vi "Time domain Tx-TF Correction.vi"(7 "Normalize to TF":bool=TRUE, 10 "window":T1=1 items=["Rectangle"=0, "Hanning"=1, "Hamming"=2, "Blackman-Harris"=3, "Exact Blackman"=4, "Blackman"=5, "Flat Top"=6, "4 Term B-Harris "=7, "7 Term B-Harris"=8, "Low Sidelobe"=9, "Blackman Nuttall"=11, "Triangle"=30, "Bartlett-Hanning"=31, "Bohman"=32, "Parzen"=33, "Welch"=34, "Kaiser"=60, "Dolph-Chebyshev"=61, "Gaussian"=62], 11 "Tx Waveform":waveform(dbl)={"t0"=timestamp(3728232981.5205336 s since 1904-01-01), "dt"=9.9999999999997e-07, "Y"=array[20000 elements], "attributes"=variant("NI_ChannelName"=variant(string "H1/ai7"), "NI_UnitDescription"=variant(string "Volts"))}) -> (0 "Rx FFT _NoCorrect":cluster{"f0":dbl, "df":dbl, "magnitude":dbl[]}(graph), 1 "Waveform Graph":cluster{"f0":dbl, "df":dbl, "magnitude":dbl[]}(graph), 2 "TF units from loaded file":string, 3 "TF Corr Rx FFT complex":T2, 4 "IMon magnitude":dbl, 6 "THD":dbl)   [LabVIEW 2021]
uses:
  <vilib>/Analysis/4window.llb/windowTd.ctl
  <vilib>/measure/maspectr.llb/Power Spectrum and PSD Export Mode.ctl
  <vilib>/Analysis/2dsp.llb/Inverse Real FFT.vi
  <vilib>/measure/maspectr.llb/FFT Spectrum (Mag-Phase) for 1 Chan.vi
  <vilib>/measure/maspectr.llb/FFT Power Spectrum and PSD for 1 Chan.vi
  MPS_Labview/MPS_global_variables.vi
  <vilib>/measure/NI_MAPro.lvlib
  <vilib>/Analysis/NI_AALPro.lvlib
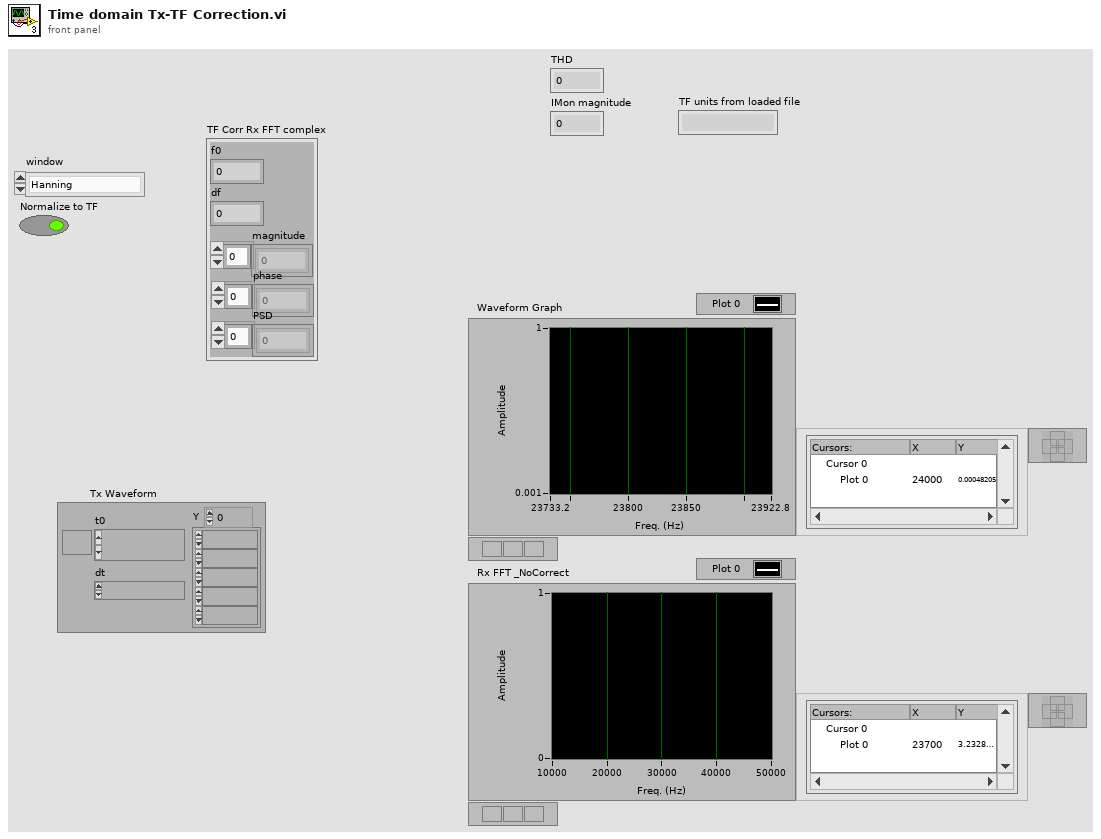
[diagram p1: front panel]
types:
  T1 = typedef "NI_AALPro.lvlib/windowTd.ctl" = u32
  T2 = cluster{"f0":dbl, "df":dbl, "magnitude":dbl[], "phase":dbl[], "PSD":dbl[]}
  T3 = cluster{"sample rate":dbl, "Transmit frequency":dbl, "Transmit amplitude":dbl, "sample rate digital out":dbl, "TX cycles":i32, "sample rate DAQ1":dbl, "Receive frequency":dbl, "Receive range":dbl, "TX harmonics":dbl[]}
  T4 = typedef "NI_MAPro.lvlib/Power Spectrum and PSD Export Mode.ctl" = u16
  T5 = cluster{"sample rate":dbl, "Tx freq":dbl, "Tx amp":dbl, "Tx cycles\nSpectroscopy":dbl, "Bias amp":dbl, "Bias freq":dbl, "Receive range":dbl, "Bias Periods\nMagnetometry":dbl, "Tx Freq Division Factor":dbl, "Drive Periods per Bias":dbl, "TX harmonics":dbl[]}
  T6 = cluster{"f0":dbl, "df":dbl, "magnitude":dbl[], "phase":dbl[], dbl[]}
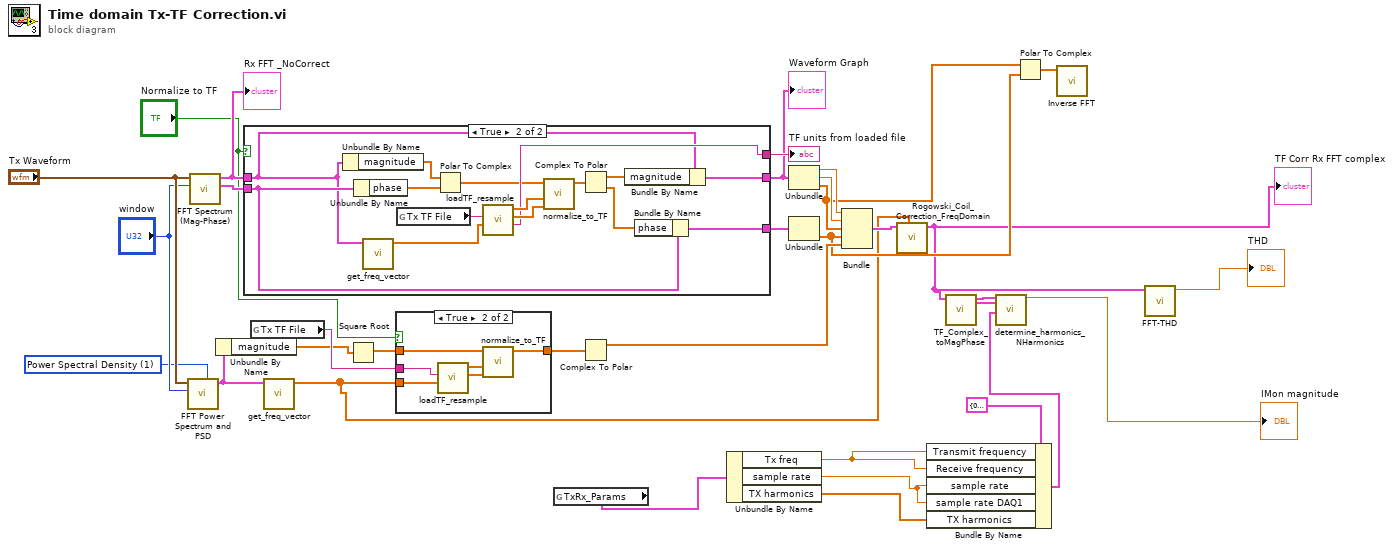
[diagram p0: block diagram]
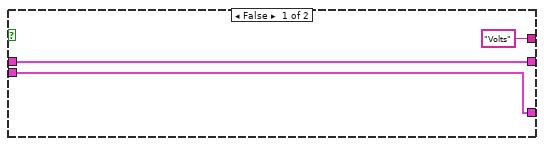
[diagram p3: hidden frame]
diagram:
  w23 = T4 1 items=["Power Spectrum", "Power Spectral Density"] ("export mode")
  n1 = call-poly <vilib>:"FFT Power Spectrum and PSD.vi"("export mode"=w23, "window"="window", "time signal"="Tx Waveform") -> ("Power Spectrum / PSD"=w26:cluster{"f0":dbl, "df":dbl, "magnitude":dbl[]})  [unwired: 5 in, 3 out]
  n2 = call-poly <vilib>:"FFT Spectrum (Mag-Phase).vi"("window"="window", "time signal"="Tx Waveform") -> ("phase"=w33:cluster{"f0":dbl, "df":dbl, "phase":dbl[]}, "magnitude"=w31:cluster{"f0":dbl, "df":dbl, "magnitude":dbl[]})  [unwired: 5 in, 3 out]
  "Rx FFT _NoCorrect" <- w31
  n3 = Unbundle By Name(w26) -> ("magnitude"=w20:dbl[])
  n4 = case shown="True" "Normalize to TF" {
    tunnel: w33 -> [w35 w46]
    tunnel: ["Volts" ("TF units from loaded file") w43] -> w32
    tunnel: w31 -> [w36 w37]
    tunnel: [w36 w39] -> w15
    tunnel: [w35 w38] -> w14
    frame False {
    }
    frame True {
      n5 = Unbundle By Name(w37) -> ("magnitude"=w48:dbl[])
      n6 = Unbundle By Name(w46) -> ("phase"=w47:dbl[])
      n7 = call "get_freq_vector.vi"("FFT magnitude"=w37) -> ("Freq array"=w49:dbl[])  [unwired: 10 in]
      n8 = global read "MPS_global_variables.vi" "Tx TF File"() -> (w44:string)
      n9 = Polar To Complex(1:w47, 2:w48) -> (0:w41:cdb[])
      n10 = call "loadTF_resample.vi"("desired freqs"=w49, "mat file name"=w44) -> ("TF units from loaded file"=w43:string, "output TF phase"=w51:dbl[], "output TF mag"=w50:dbl[])  [unwired: 7 in]
      n11 = call "normalize_to_TF.vi"("TF phase"=w51, "TF mag"=w50, "signal (can be complex)"=w41) -> ("signal normalized to TF (can be complex)"=w40:cdb[])  [unwired: 8 in]
      n12 = Complex To Polar(r * e^(i*theta)=w40) -> (r=w42:dbl[], theta=w45:dbl[])
      n13 = Bundle By Name(cluster=w37, "magnitude"=w42) -> (w39:cluster{"f0":dbl, "df":dbl, "magnitude":dbl[]})
      n14 = Bundle By Name(cluster=w46, "phase"=w45) -> (w38:cluster{"f0":dbl, "df":dbl, "phase":dbl[]})
    }
  }
  "TF units from loaded file" <- w32
  "Waveform Graph" <- w15
  n15 = global read "MPS_global_variables.vi" "Tx TF File"() -> (w27:string)
  n16 = call "get_freq_vector.vi"("FFT magnitude"=w26) -> ("Freq array"=w1:dbl[])  [unwired: 10 in]
  n17 = Square Root(x=w20) -> (sqrt(x)=w21:dbl[])
  n18 = case shown="True" "Normalize to TF" {
    tunnel: [w52 w58] -> w28
    tunnel: w27 -> [_ w57]
    tunnel: w1 -> [_ w56]
    tunnel: w21 -> [w52 w53]
    frame False {
    }
    frame True {
      n19 = call "loadTF_resample.vi"("desired freqs"=w56, "mat file name"=w57) -> ("output TF phase"=w54:dbl[], "output TF mag"=w55:dbl[])  [unwired: 7 in, 1 out]
      n20 = call "normalize_to_TF.vi"("TF phase"=w54, "TF mag"=w55, "signal (can be complex)"=w53) -> ("signal normalized to TF (can be complex)"=w58:cdb[])  [unwired: 8 in]
    }
  }
  n21 = global read "MPS_global_variables.vi" "TxRx_Params"() -> (w13:T5)
  n22 = Complex To Polar(r * e^(i*theta)=w28) -> (r=w25:dbl[])  [unwired: 1 out]
  n23 = Unbundle By Name(w13) -> ("Tx freq"=w11:dbl, "sample rate"=w10:dbl, "TX harmonics"=w9:dbl[])
  n24 = Unbundle(w15) -> ("f0"=w19:dbl, "df"=w30:dbl, "magnitude"=w18:dbl[])
  n25 = Unbundle(w14) -> ("phase"=w17:dbl[])  [unwired: 2 out]
  n26 = Bundle("f0"=w19, "df"=w30, "magnitude"=w18, "phase"=w17, w25) -> (w5:T6)  [unwired: 1 in]
  n27 = call "Rogowski_Coil_Correction_FreqDomain.vi"("Freq array"=w1, "Raw IMon FFT"=w5) -> ("TF Corr IMon FFT"=w4:T2)  [unwired: 8 in, 1 out]
  "TF Corr Rx FFT complex" <- w4
  n28 = Bundle By Name(cluster=T3 {"sample rate"=0.0, "Transmit frequency"=0.0, "Transmit amplitude"=0.0, "sample rate digital out"=0.0, "TX cycles"=0, "sample rate DAQ1"=0.0, "Receive frequency"=0.0, "Receive range"=0.0, "TX harmonics"=[]} ("TxRxParams"), "Transmit frequency"=w11, "Receive frequency"=w11, "sample rate"=w10, "sample rate DAQ1"=w10, "TX harmonics"=w9) -> (w8:T3)
  n29 = call "TF_Complex_toMagPhase.vi"("TF Corr Rx FFT Mag"=w4) -> ("TF Phase"=w2:cluster{"f0":dbl, "df":dbl, "magnitude":dbl[]}, "TF Mag"=w3:cluster{"f0":dbl, "df":dbl, "magnitude":dbl[]})  [unwired: 4 in, 5 out]
  n30 = call "determine_harmonics_NHarmonics.vi"("FFT magnitude"=w3, "FFT phase"=w2, "TxRxParams"=w8) -> ("RX magnitude"=→"IMon magnitude":dbl)  [unwired: 11 in, 5 out]
  n31 = Polar To Complex(1:w17, 2:w18) -> (0:w16:cdb[])
  n32 = call-poly <vilib>:"Inverse FFT.vi"("FFT {X}"=w16) -> ()  [unwired: 9 in, 2 out]
  n33 = call "FFT-THD.vi"("TF Corr IMon FFT"=w4) -> ("THD"=→"THD":dbl)  [unwired: 10 in]
